vi "DB - [Config].[TableGroup].vi"(4 "Application":string, 5 "Table Group Enum":T1, 6 "[Description]":string, 7 "DB Connection":T3={"Open"=TRUE, "Close"=TRUE}, 8 "error in (no error)":errorcluster, 9 "DB.Config.TableGroup":string="SRTRS.Config.TableGroup", 10 "DB.Config.TableGroupType":string="SRTRS.Config.TableGroupType", 11 "connection reference":T2) -> (0 "SUMMARY":errorcluster, 2 "data":string[](array[string]), 3 "connection reference":T2)   [LabVIEW 2013]
uses:
  <vilib>/addons/database/Connection.llb/Conn ObjectReference.ctl
  Controls/DB - OpenClose.ctl
  Controls/DB - Table Group Enum.ctl
  <vilib>/addons/database/Connection.llb/Conn Execute.vi
  <vilib>/addons/database/Recordset.llb/Rec Fetch Recordset Data (R).vi
  <vilib>/addons/database/Recordset.llb/Rec Destroy - Connection.vi
  Controls/Global SRTRS.vi
  Controls/Global CMS.vi
  Controls/Global AMS.vi
  <vilib>/addons/database/Connection.llb/DB Tools Open Connec (String).vi
  <vilib>/addons/database/_DB Variant To Data/Database Variant To Data.xnode
  <vilib>/addons/database/NI_Database_API.lvlib
panel:
  out "SQL Statement":string
  out "Connection Information":T4={"Connection "="SQL Server 32bit HPEnvy", "Username"="admin", "Password"="admin123"}
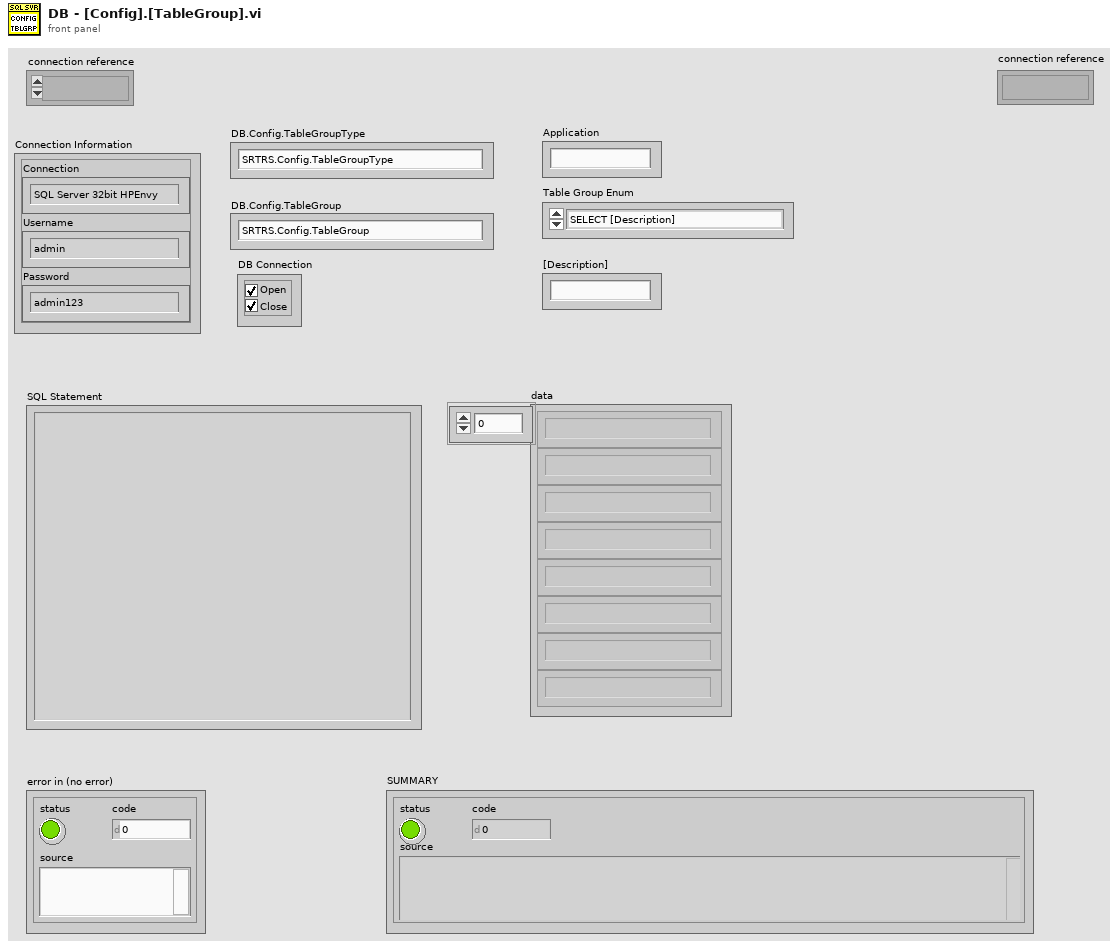
[diagram p1: front panel]
types:
  T1 = typedef "DB - Table Group Enum.ctl" = enum16{"SELECT [Description]", "SELECT [TableGroupId]"}
  T2 = typedef "NI_Database_API.lvlib/Conn ObjectReference.ctl" = refnum<k1>
  T3 = typedef "DB - OpenClose.ctl" = cluster{"Open":bool, "Close":bool}
  T4 = cluster{"Connection ":string, "Username":string, "Password":string}
  T5 = typedef "Enum - InteractiveMode-SubVIMode.ctl" = enum16{"Interactive", "subVI Mode"}
  T6 = typedef "DB - DB.Schema.Table.ctl" = cluster{"DB":string, "Schema":string, "Table":string}
  T7 = typedef "Connection Information Cluster.ctl" = cluster{"Connection ":string, "Username":string, "Password":string}
  T8 = typedef "NI_Database_API.lvlib/Rec ObjectReference.ctl" = refnum<k1>
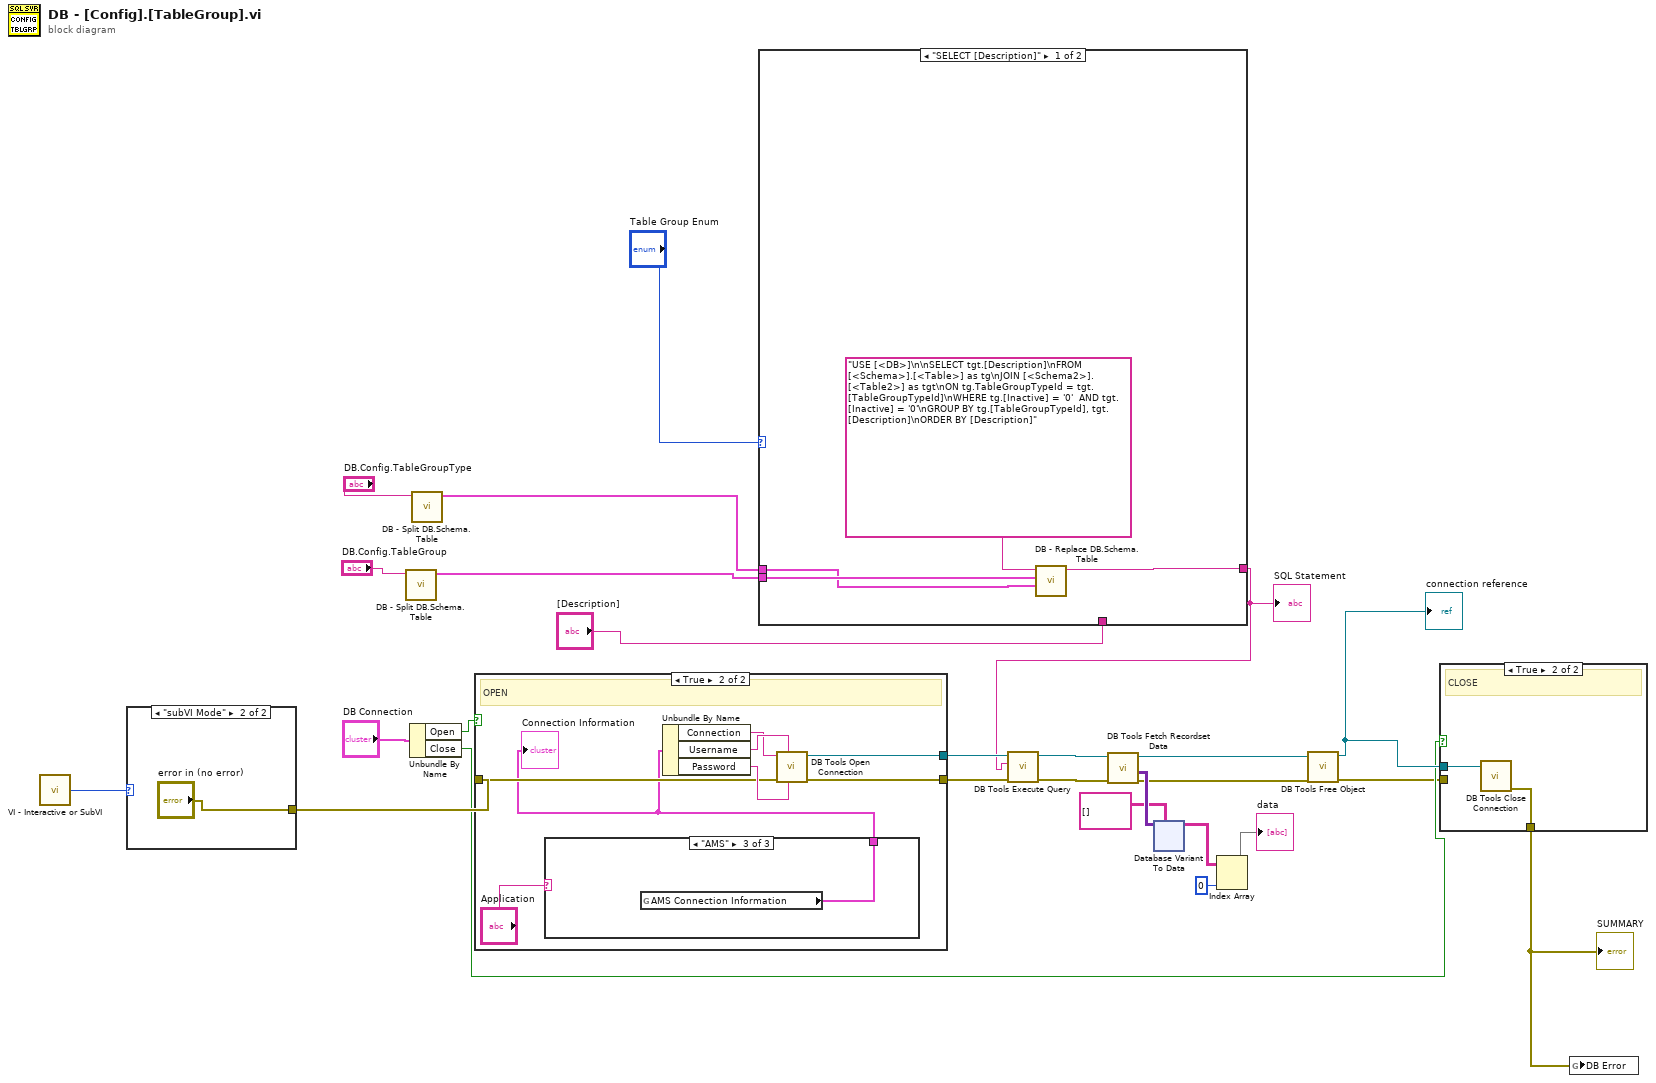
[diagram p0: block diagram]
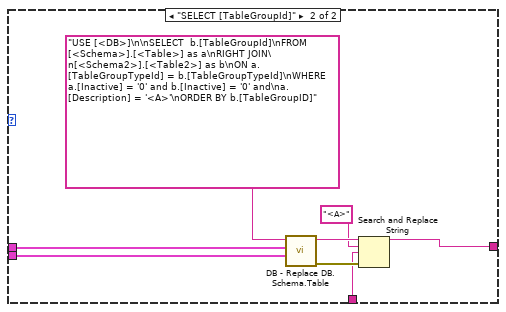
[diagram p2: hidden frame]
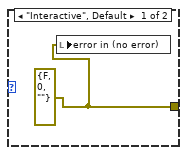
[diagram p4: hidden frame]
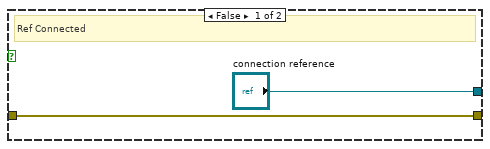
[diagram p5: hidden frame]
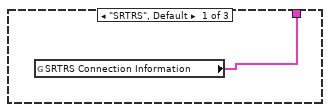
[diagram p6: hidden frame]
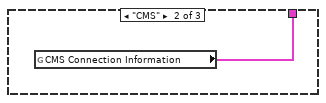
[diagram p7: hidden frame]
diagram:
  n1 = call "VI - Interactive or SubVI.vi"() -> ("Mode"=w24:T5)  [unwired: 5 in]
  n2 = case shown="\"subVI Mode\"" w24 {
    tunnel: [w27 "error in (no error)"] -> w23
    frame "Interactive", Default {
      w27 = errorcluster {"status"=FALSE, "code"=0, "source"=""} ("error in (no error)")
      n3 = local write "error in (no error)"(w27) -> ()
    }
    frame "subVI Mode" {
    }
  }
  n4 = call "DB - Split DB.Schema.Table.vi"("DB.Schema.Table"="DB.Config.TableGroup") -> ("DB.Schema.Table"=w7:T6)  [unwired: 10 in]
  n5 = Unbundle By Name("DB Connection") -> ("Open"=w25:bool, "Close"=w12:bool)
  n6 = call "DB - Split DB.Schema.Table.vi"("DB.Schema.Table"="DB.Config.TableGroupType") -> ("DB.Schema.Table"=w8:T6)  [unwired: 10 in]
  n7 = case shown="True" w25 {
    tunnel: ["connection reference" w35] -> w16
    tunnel: w23 -> [w29 w34]
    tunnel: [w29 w33] -> w15
    frame False {
      # "Ref Connected"
    }
    frame True {
      # "OPEN"
      n8 = case shown="\"AMS\"" "Application" {
        tunnel: [w39 w40 w41] -> w31
        frame "SRTRS", Default {
          n9 = global read "Global SRTRS.vi" "SRTRS Connection Information"() -> (w39:T7)
        }
        frame "CMS" {
          n10 = global read "Global CMS.vi" "CMS Connection Information"() -> (w40:T7)
        }
        frame "AMS" {
          n11 = global read "Global AMS.vi" "AMS Connection Information"() -> (w41:T7)
        }
      }
      "Connection Information" <- w31
      n12 = Unbundle By Name(w31) -> ("Connection"=w37:string, "Username"=w38:string, "Password"=w36:string)
      n13 = call-poly <vilib>:"DB Tools Open Connection.vi"("password"=w36, "userID"=w38, "error in (no error)"=w34, "connection information"=w37) -> ("error out"=w33:errorcluster, "connection reference"=w35:T2)  [unwired: 4 in]
    }
  }
  n14 = case shown="\"SELECT [Description]\"" "Table Group Enum" {
    tunnel: w8 -> [w42 w52]
    tunnel: w7 -> [w43 w51]
    tunnel: [w44 w49] -> w6
    tunnel: "[Description]" -> [_ w46]
    frame "SELECT [Description]" {
      n15 = call "DB - Replace DB.Schema.Table.vi"("DB.Schema.Table 2"=w42, "DB.Schema.Table"=w43, "string in"="USE [<DB>]\n\nSELECT tgt.[Description]\nFROM [<Schema>].[<Table>] as tg\nJOIN [<Schema2>].[<Table2>] as tgt\nON tg.TableGroupTypeId = tgt.[TableGroupTypeId]\nWHERE tg.[Inactive] = '0'  AND tgt.[Inactive] = '0'\nGROUP BY tg.[TableGroupTypeId], tgt.[Description]\nORDER BY [Description]" ("SQL query")) -> ("string out"=w44:string)  [unwired: 7 in, 1 out]
    }
    frame "SELECT [TableGroupId]" {
      n16 = call "DB - Replace DB.Schema.Table.vi"("DB.Schema.Table 2"=w51, "DB.Schema.Table"=w52, "string in"="USE [<DB>]\n\nSELECT  b.[TableGroupId]\nFROM [<Schema>].[<Table>] as a\nRIGHT JOIN\n[<Schema2>].[<Table2>] as b\nON a.[TableGroupTypeId] = b.[TableGroupTypeId]\nWHERE a.[Inactive] = '0' and b.[Inactive] = '0' and\na.[Description] = '<A>'\nORDER BY b.[TableGroupID]" ("SQL query")) -> ("error out"=w48:errorcluster, "string out"=w50:string)  [unwired: 7 in]
      n17 = Search and Replace String(input string=w50, search string="<A>", replace string=w46, error in=w48) -> (result string=w49:string)  [unwired: 4 in, 3 out]
    }
  }
  "SQL Statement" <- w6
  n18 = call-poly <vilib>:"DB Tools Execute Query.vi"("error in (no error)"=w15, "SQL query"=w6, "connection reference"=w16) -> ("error out"=w22:errorcluster, "recordset reference"=w21:T8)  [unwired: 5 in]
  n19 = call-poly <vilib>:"DB Tools Fetch Recordset Data.vi"("error in (no error)"=w22, "recordset reference"=w21) -> ("error out"=w17:errorcluster, "recordset data"=w20:variant[][], "recordset reference out"=w18:T8)  [unwired: 3 in]
  n20 = xnode "Database Variant To Data"("database variant"=w20, "type"=string[][] []) -> ("data"=w3:string[][])  [unwired: 1 in, 1 out]
  n21 = Index Array(array=w3, index (col)=0 ("disabled index (col)")) -> (element=→"data":string[])  [unwired: 1 in]
  n22 = call-poly <vilib>:"DB Tools Free Object.vi"("error in (no error)"=w17, "recordset reference"=w18) -> ("error out"=w11:errorcluster, "connection reference"=w13:T2)  [unwired: 8 in]
  "connection reference" <- w13
  n23 = case shown="True" w12 {
    tunnel: [w54 w55] -> w14
    tunnel: w13 -> [_ w56]
    tunnel: w11 -> [w54 _]
    frame False {
      # "Ref Connected"
    }
    frame True {
      # "CLOSE"
      n24 = call <vilib>:"DB Tools Close Connection.vi"("connection reference"=w56) -> ("error out"=w55:errorcluster)  [unwired: 6 in]
    }
  }
  "SUMMARY" <- w14
  n25 = global write "Global SRTRS.vi" "DB Error"(w14) -> ()
